vi "Replace_Shortcut.vi"(8 "error in (no error)":errorcluster, 9 "shortcut":T1, 10 "index":i32, 11 "Installer in":refnum<class "Installer.lvclass">) -> (0 "error out":errorcluster, 3 "Installer out":refnum<class "Installer.lvclass">)   [LabVIEW 2020, in "Installer.lvclass"]
uses:
  <vilib>/AppBuilder/IB_Classes/Installer/Installer.lvclass
  <vilib>/AppBuilder/IB_Classes/Installer/Installer.lvclass/Installer.ctl
  <resource>/Framework/Providers/Builds/Installer/CDK_sTypeDef_ShortcutAddress.ctl
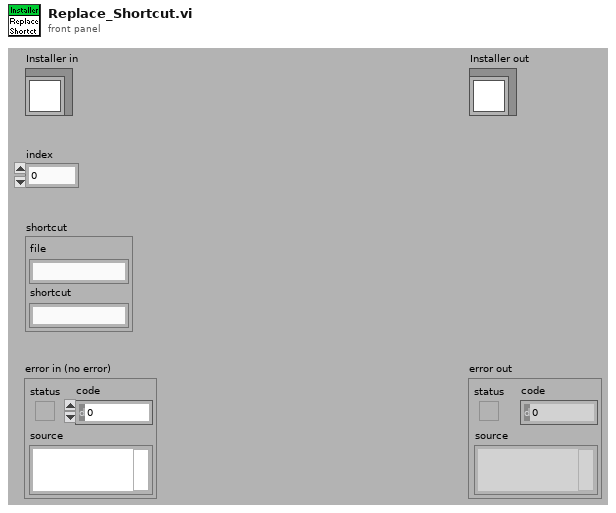
[diagram p1: front panel]
types:
  T1 = typedef "CDK_sTypeDef_ShortcutAddress.ctl" = cluster{"file":string, "shortcut":string}
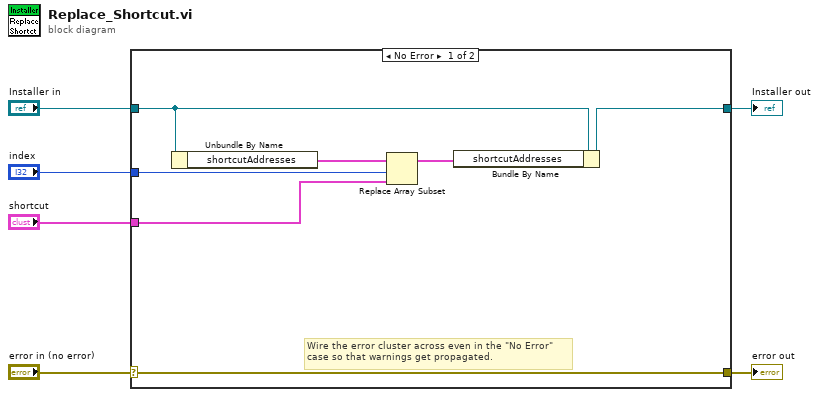
[diagram p0: block diagram]
diagram:
  n1 = case shown="No Error" "error in (no error)" {
    selector: "error in (no error)" -> [w13 w15]
    tunnel: [w13 w15] -> w5
    tunnel: [w8 w14] -> w3
    tunnel: "Installer in" -> [w9 w14]
    tunnel: "index" -> [w11 _]
    tunnel: "shortcut" -> [w10 _]
    frame No Error {
      # "Wire the error cluster across even in the \"No Error\"\ncase so that warnings get propagated."
      n2 = Unbundle By Name(w9) -> ("shortcutAddresses"=w12:T1[])
      n3 = Replace Array Subset(array=w12, new element=w10, index=w11) -> (w7:T1[])
      n4 = Bundle By Name(cluster=w9, "shortcutAddresses"=w7) -> (w8:refnum<class "Installer.lvclass">)
    }
    frame Error {
    }
  }
  "error out" <- w5
  "Installer out" <- w3
